vi "classify error.vi"(8 "error to classify":errorcluster, 10 "attempt recovery?":bool, 11 "module in":refnum<class "TBM module execution interface.lvclass">) -> (0 "classified error":errorcluster, 2 "error classification":T1, 3 "module out":refnum<class "TBM module execution interface.lvclass">)   [LabVIEW 2013, in "TBM module execution interface.lvclass"]
doc: "Allows a module to classify an error generated at any point during execution. This <b>error classification</b> can then be used by calling code to determine if execution can continue. In addition, this function can be used to allow a component to clear an error, convert an error to a warning, or attempt to recover from an error. Recovery may be attempted only if <b>attempt recovery?</b> is true."
uses:
  TBM module execution interface.lvclass
  error classification.ctl
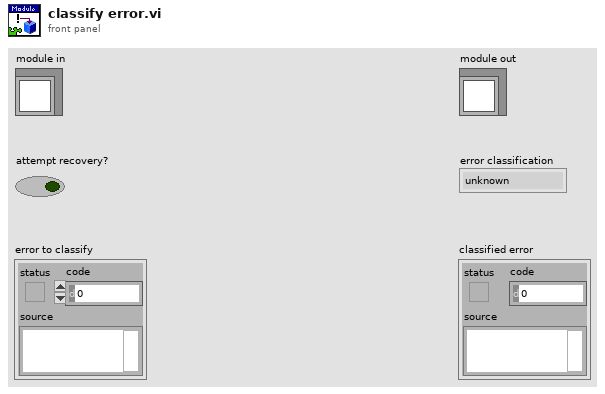
[diagram p1: front panel]
types:
  T1 = typedef "TBM module execution interface.lvclass/error classification.ctl" = enum16{"unknown", "none", "trivial", "recoverable", "critical"}
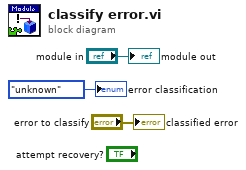
[diagram p0: block diagram]
diagram:
  "module out" <- "module in"
  "error classification" <- error_classification."unknown" ("error classification")
  "classified error" <- "error to classify"
